vi "Do Draw.vi"(9 "color":u32(colorbox), 10 "picture in":picture, 11 "Draw Message":refnum<class "Draw Message.lvclass">) -> (2 "picture out":picture)   [LabVIEW 2019, in "Draw Messages.lvlib" / "Draw Message.lvclass"]
doc: "Draw whatever the message needs to draw into the picture."
uses:
  Draw Message.lvclass
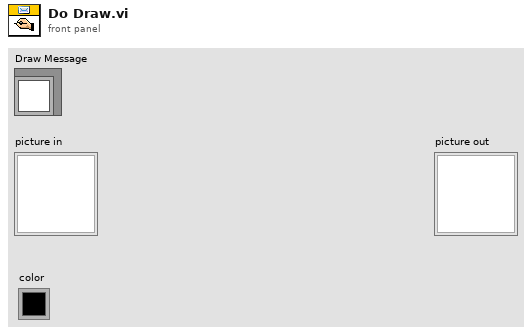
[diagram p1: front panel]
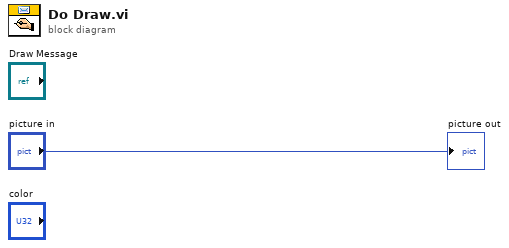
[diagram p0: block diagram]
diagram:
  "picture out" <- "picture in"
